vi "Main.vi"() -> ()   [LabVIEW 2014]
doc: "The boiler controller allows a user to start and shut down a boiler.\n\nUse the Reset, Start, and Light Pilot controls to sequentially start the boiler. \nUse the Fuel Control Valve to change the flow of fuel into the boiler. \nUse the Stop Boiler button to shut down the boiler. \nTo shut down the system or in the event of an emergency, use the Emergency Stop button to close the application completely."
uses:
  controls/MHL Data.ctl
  controls/MHL UI Data.ctl
  controls/MHL Status.ctl
  controls/MHL References.ctl
  controls/MHL Configuration.ctl
  support/Boiler System Globals.vi
  <vilib>/Utility/error.llb/Error Cluster From Error Code.vi
  <vilib>/ErrorRing/Error Ring.xnode
  support/Message Queue/Message Queue.lvlib
  support/User Event - Stop/User Event - Stop.lvlib
  Controller/Controller.lvlib
  Boiler/Boiler.lvlib
panel:
  in  "Fuel Control Valve":u32(slide) min=10 max=75 scale=10.0..75.0
  in  "Stop Boiler":bool
  in  "Light Pilot":bool
  out "Forced Draft Fan":bool
  out "Pilot":bool
  out "Pilot Gas Valve":bool
  out "Primary Fan":bool
  out "Status":string
  in  "Start":bool
  in  "Reset":bool
  in  "Emergency Stop":bool
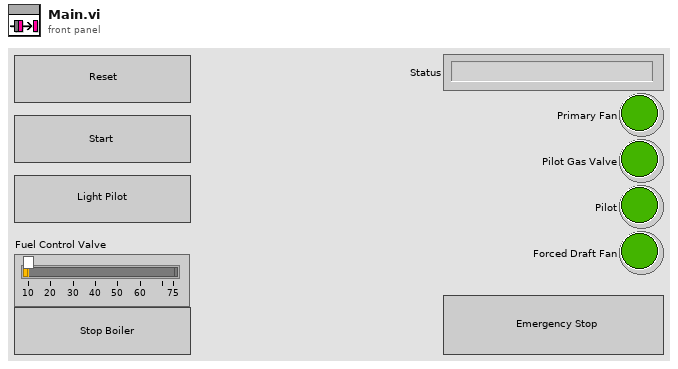
[diagram p1: front panel]
types:
  T1 = typedef "MHL Data.ctl" = cluster{"MHL User Interface Data":T2, "MHL References":T4, "MHL Configuration":T5}
  T2 = typedef "MHL UI Data.ctl" = cluster{"Status":string, "Fuel Control Valve":u32, "Primary Fan":bool, "Pilot Gas Valve":bool, "Pilot":bool, "Forced Draft Fan":bool, "MHL Status":T3}
  T3 = typedef "MHL Status.ctl" = enum16{"Lockout", "Ready", "Pre-Purge", "Pre-Purge Complete", "Pilot On", "Boiler Running", "Shutdown", "Purge"}
  T4 = typedef "MHL References.ctl" = cluster{"Reset Ref":refnum<vi>, "Start Ref":refnum<vi>, "Light Pilot Ref":refnum<vi>, "Stop Boiler Ref":refnum<vi>, "Fuel Control Valve Ref":refnum<vi>}
  T5 = typedef "MHL Configuration.ctl" = cluster{"Fuel Control Valve Maximum":dbl, "Fuel Control Valve Minimum":dbl}
  T6 = typedef "Configuration Data.ctl" = cluster{"MHL Configuration":T5, "Controller Configuration":T7, "Boiler Configuration":T8}
  T7 = typedef "Controller.lvlib/Controller Configuration.ctl" = cluster{"Purge Time":u32, "Flame Threshold":u32}
  T8 = typedef "Boiler.lvlib/Boiler Configuration.ctl" = cluster{"Pilot Increment (ms)":u32, "Pilot Decrement (ms)":u32}
  T9 = typedef "Notifiers.ctl" = cluster{"Handshake":refnum<notifier>, "Flame Level":refnum<notifier>, "Controller Exit":refnum<notifier>, "Boiler Exit":refnum<notifier>}
  T10 = typedef "Message Queue.lvlib/All Message Queues.ctl" = cluster{"MHL":refnum<queue>, "Boiler Controller":refnum<queue>, "Boiler":refnum<queue>}
  T11 = enum16{"open", "replace", "create", "open or create", "replace or create", "replace or create with confirmation"}
  T12 = enum32{"invalid app kind", "Development System", "Run Time System", "Student Edition", "Embedded LabVIEW", "Evaluation", "Custom"}
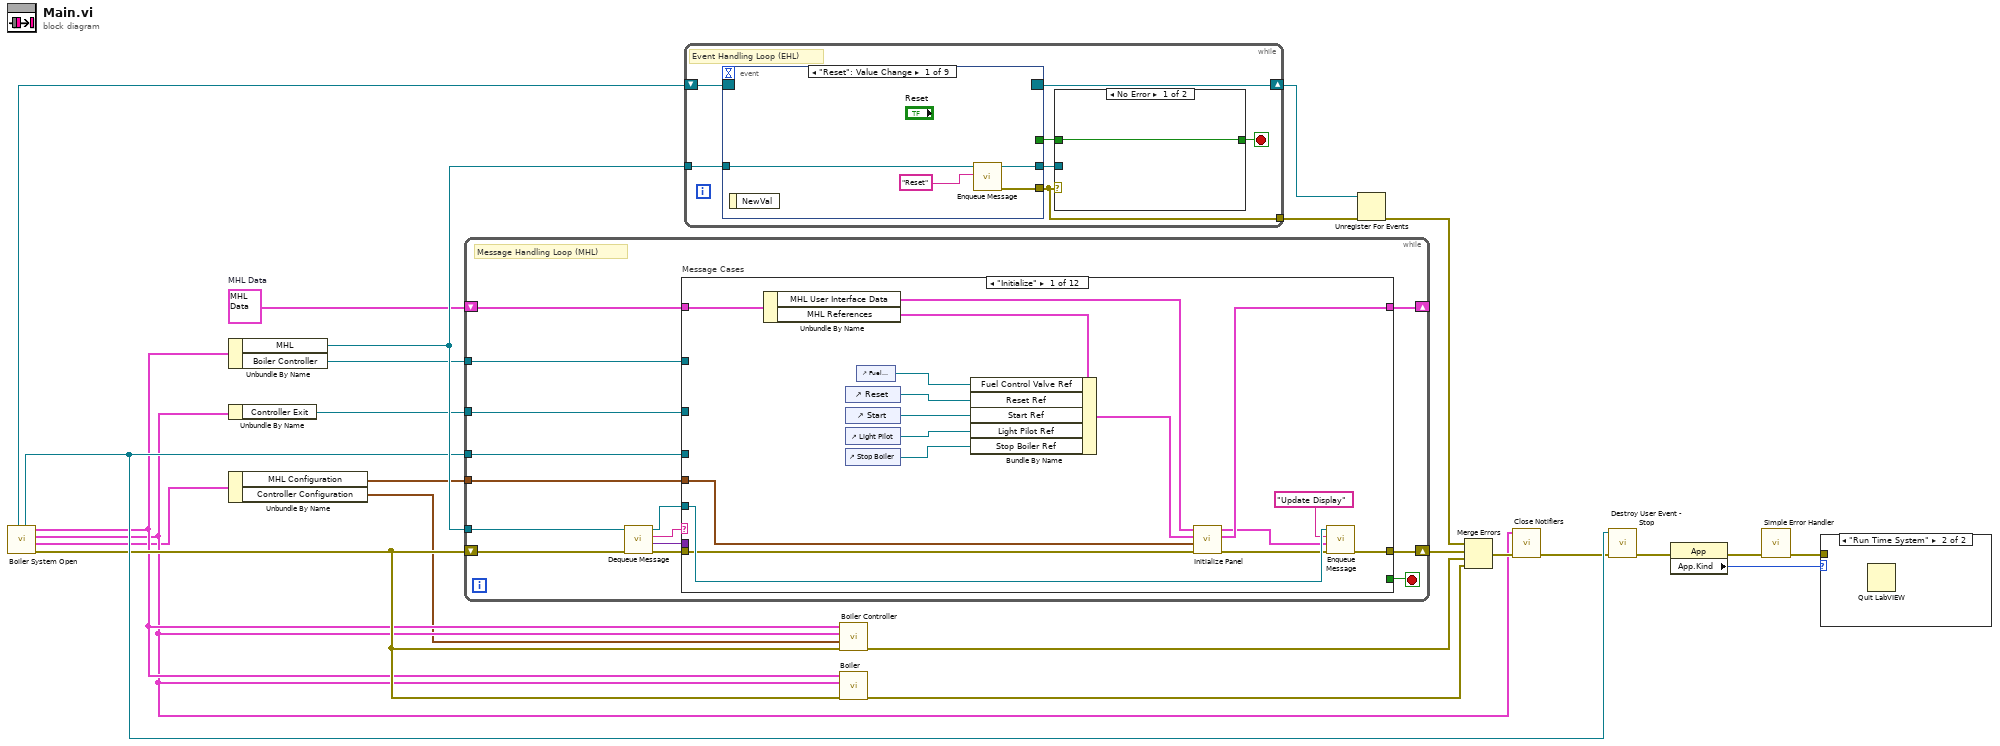
[diagram p0: block diagram]
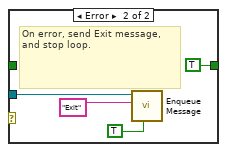
[diagram p3: hidden frame]
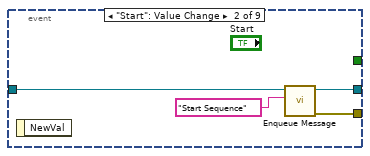
[diagram p4: hidden frame]
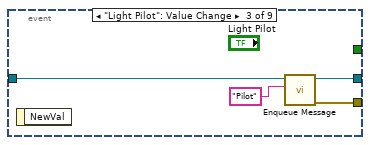
[diagram p5: hidden frame]
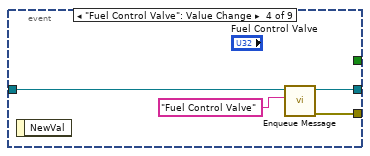
[diagram p6: hidden frame]
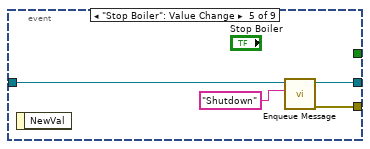
[diagram p7: hidden frame]
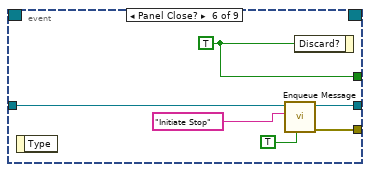
[diagram p8: hidden frame]
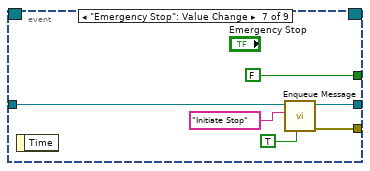
[diagram p9: hidden frame]
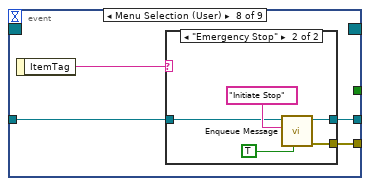
[diagram p10: hidden frame]
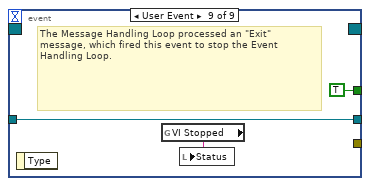
[diagram p12: hidden frame]
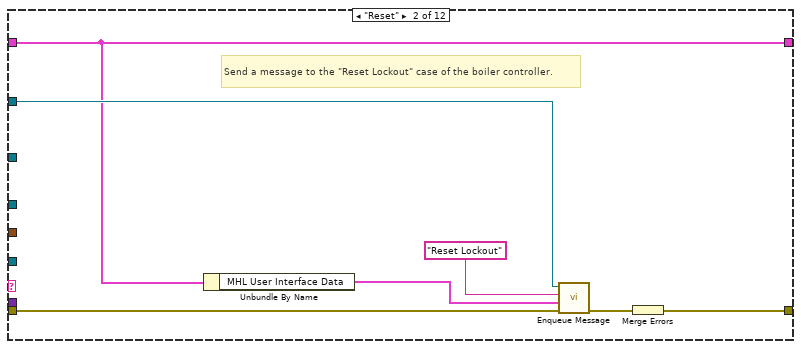
[diagram p13: hidden frame]
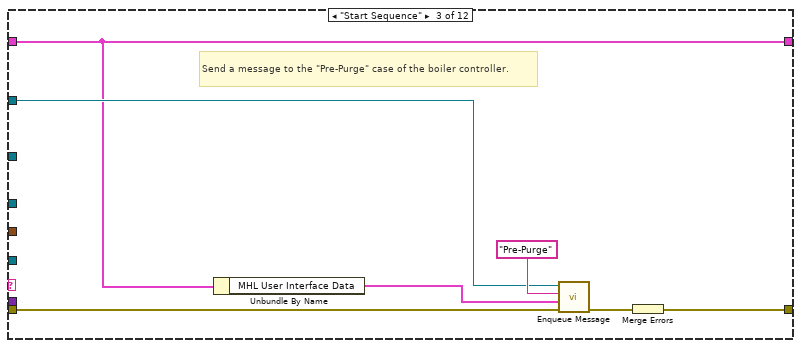
[diagram p14: hidden frame]
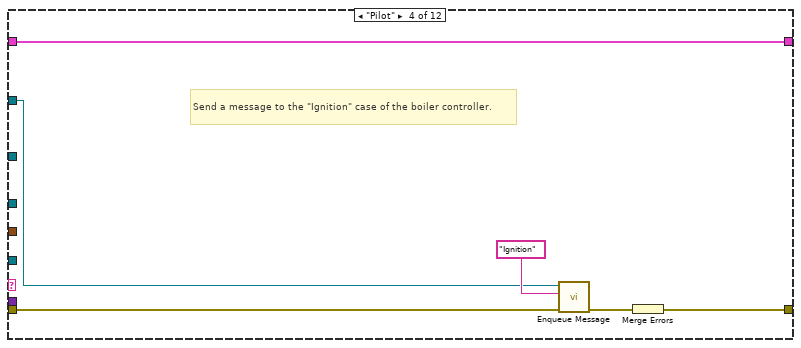
[diagram p15: hidden frame]
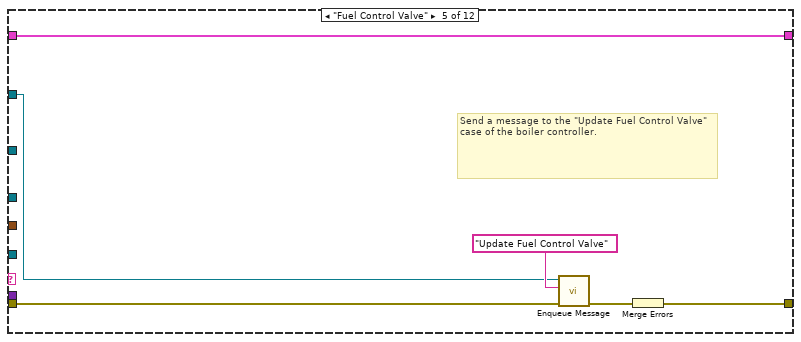
[diagram p16: hidden frame]
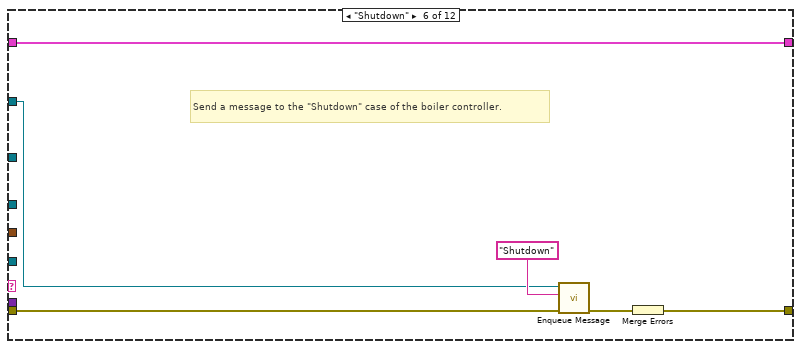
[diagram p17: hidden frame]
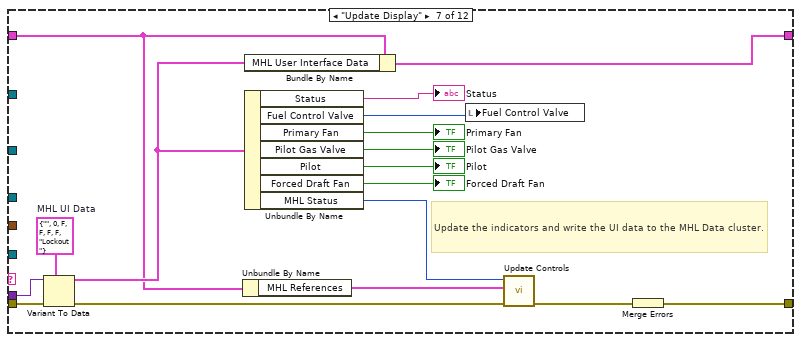
[diagram p18: hidden frame]
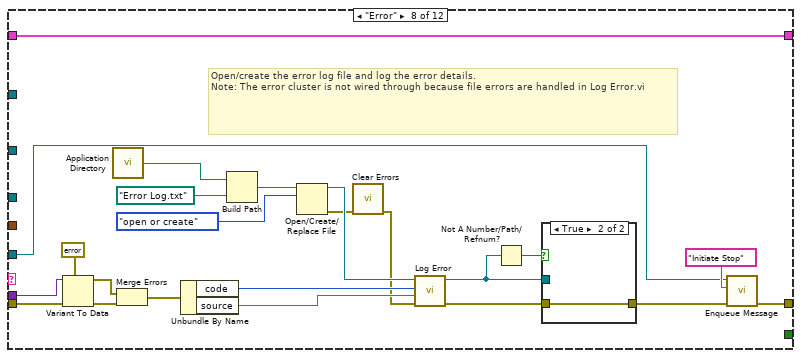
[diagram p19: hidden frame]
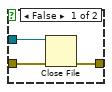
[diagram p20: hidden frame]
diagram:
  w18 = T1 {"MHL User Interface Data"={"Status"="", "Fuel Control Valve"=0, "Primary Fan"=FALSE, "Pilot Gas Valve"=FALSE, "Pilot"=FALSE, "Forced Draft Fan"=FALSE, "MHL Status"=enum."Lockout"}, "MHL References"={"Reset Ref"=refnum, "Start Ref"=refnum, "Light Pilot Ref"=refnum, "Stop Boiler Ref"=refnum, "Fuel Control Valve Ref"=refnum}, "MHL Configuration"={"Fuel Control Valve Maximum"=0.0, "Fuel Control Valve Minimum"=0.0}}  # MHL Data
  n1 = call "Boiler System Open.vi"() -> ("error out"=w9:errorcluster, "Configuration Data"=w3:T6, "Notifiers"=w4:T9, "Message Queues"=w8:T10, "User Event - Stop"=w11:refnum<user-event>, "Stop Event Registration Refnum"=w12:refnum<event-registration>)  [unwired: 6 in]
  n2 = Unbundle By Name(w8) -> ("MHL"=w23:refnum<queue>, "Boiler Controller"=w16:refnum<queue>)
  n3 = Unbundle By Name(w4) -> ("Controller Exit"=w10:refnum<notifier>)
  n4 = Unbundle By Name(w3) -> ("MHL Configuration"=w2:T5, "Controller Configuration"=w1:T7)
  n5 = while {
    tunnel: w23 -> [w28]
    shift-right: [w37] -> _
    shift-left: w18 -> [w38]
    tunnel: w11 -> [w34]
    shift-right: [w35] -> w24
    shift-left: w9 -> [w33]
    tunnel: w16 -> [w27]
    tunnel: w10 -> [w26]
    tunnel: w2 -> [w25]
    stop <- w36 stop-if-true
    # "Message Handling Loop (MHL)"
    n6 = call "Dequeue Message.vi"("error in (no error)"=w33, "Message Queue"=w28) -> ("error out"=w32:errorcluster, "Message Data"=w30:variant, "Message"=w31:string, "dup Message Queue"=w29:refnum<queue>)  [unwired: 6 in]
    n7 = case "Message Cases" shown="\"Initialize\"" w31 {
      selector: w31 -> [_ _ _ _ _ _ _ _ _ _ _ w165]
      tunnel: w29 -> [w48 _ _ _ _ _ _ w113 w134 w141 w163 _]
      tunnel: w32 -> [w42 w61 w68 w73 w76 w85 w103 w111 w139 w143 w156 _]
      tunnel: [w49 w62 w69 w74 w81 w86 w104 w109 w136 w142 w159 w164] -> w35
      tunnel: w38 -> [w50 w57 w64 w75 w77 w87 w89 w127 w138 w147 w162 w166]
      tunnel: [w40 w57 w64 w75 w77 w87 w93 w127 w138 w147 w162 w166] -> w37
      tunnel: [_ _ _ _ _ _ _ _ _ _ TRUE _] -> w36
      tunnel: w30 -> [_ _ _ _ _ _ w102 w110 _ _ _ _]
      tunnel: w34 -> [_ _ _ _ _ _ _ _ _ _ w158 _]
      tunnel: w27 -> [_ w58 w65 w70 w78 w82 _ _ w135 _ _ _]
      tunnel: w26 -> [_ _ _ _ _ _ _ _ _ w140 _ _]
      tunnel: w25 -> [w46 _ _ _ _ _ _ _ _ _ _ _]
      frame "Initialize" {
        n8 = Unbundle By Name(w50) -> ("MHL User Interface Data"=w43:T2, "MHL References"=w44:T4)
        n9 = control-ref of="Reset"() -> (w52:refnum<vi>)
        n10 = control-ref of="Start"() -> (w53:refnum<vi>)
        n11 = control-ref of="Light Pilot"() -> (w54:refnum<vi>)
        n12 = control-ref of="Stop Boiler"() -> (w55:refnum<vi>)
        n13 = control-ref of="Fuel Control Valve"() -> (w51:refnum<vi>)
        n14 = Bundle By Name(cluster=w44, "Fuel Control Valve Ref"=w51, "Reset Ref"=w52, "Start Ref"=w53, "Light Pilot Ref"=w54, "Stop Boiler Ref"=w55) -> (w45:T4)
        n15 = call "Initialize Panel.vi"("error in"=w42, "MHL Configuration"=w46, "MHL References"=w45, "MHL UI Data in"=w43) -> ("error out"=w41:errorcluster, "MHL Data out"=w40:T1, "MHL UI Data out"=w39:T2)  [unwired: 5 in]
        n16 = call "Enqueue Message.vi"("error in (no error)"=w41, "Message Data"=w39, "Message"="Update Display", "Message Queue"=w48) -> ("error out"=w49:errorcluster)  [unwired: 6 in, 1 out]
      }
      frame "Reset" {
        # "Send a message to the \"Reset Lockout\" case of the boiler controller."
        n17 = Unbundle By Name(w57) -> ("MHL User Interface Data"=w56:T2)
        n18 = call "Enqueue Message.vi"("error in (no error)"=w61, "Message Data"=w56, "Message"="Reset Lockout", "Message Queue"=w58) -> ("error out"=w60:errorcluster)  [unwired: 6 in, 1 out]
        n19 = Merge Errors(w60) -> (w62:errorcluster)
      }
      frame "Start Sequence" {
        # "Send a message to the \"Pre-Purge\" case of the boiler controller."
        n20 = Unbundle By Name(w64) -> ("MHL User Interface Data"=w63:T2)
        n21 = call "Enqueue Message.vi"("error in (no error)"=w68, "Message Data"=w63, "Message"="Pre-Purge", "Message Queue"=w65) -> ("error out"=w67:errorcluster)  [unwired: 6 in, 1 out]
        n22 = Merge Errors(w67) -> (w69:errorcluster)
      }
      frame "Pilot" {
        # "Send a message to the \"Ignition\" case of the boiler controller."
        n23 = call "Enqueue Message.vi"("error in (no error)"=w73, "Message"="Ignition", "Message Queue"=w70) -> ("error out"=w72:errorcluster)  [unwired: 7 in, 1 out]
        n24 = Merge Errors(w72) -> (w74:errorcluster)
      }
      frame "Fuel Control Valve" {
        # "Send a message to the \"Update Fuel Control Valve\" case of the boiler controller."
        n25 = call "Enqueue Message.vi"("error in (no error)"=w76, "Message"="Update Fuel Control Valve", "Message Queue"=w78) -> ("error out"=w80:errorcluster)  [unwired: 7 in, 1 out]
        n26 = Merge Errors(w80) -> (w81:errorcluster)
      }
      frame "Shutdown" {
        # "Send a message to the \"Shutdown\" case of the boiler controller."
        n27 = call "Enqueue Message.vi"("error in (no error)"=w85, "Message"="Shutdown", "Message Queue"=w82) -> ("error out"=w84:errorcluster)  [unwired: 7 in, 1 out]
        n28 = Merge Errors(w84) -> (w86:errorcluster)
      }
      frame "Update Display" {
        w101 = T2 {"Status"="", "Fuel Control Valve"=0, "Primary Fan"=FALSE, "Pilot Gas Valve"=FALSE, "Pilot"=FALSE, "Forced Draft Fan"=FALSE, "MHL Status"=enum."Lockout"}  # MHL UI Data
        # "Update the indicators and write the UI data to the MHL Data cluster."
        n29 = Variant To Data(error in=w103, type=w101, Variant=w102) -> (data=w94:T2, error out=w92:errorcluster)
        n30 = Unbundle By Name(w89) -> ("MHL References"=w88:T4)
        n31 = Bundle By Name(cluster=w89, "MHL User Interface Data"=w94) -> (w93:T1)
        n32 = Unbundle By Name(w94) -> ("Status"=→"Status":string, "Fuel Control Valve"=w99:u32, "Primary Fan"=→"Primary Fan":bool, "Pilot Gas Valve"=→"Pilot Gas Valve":bool, "Pilot"=→"Pilot":bool, "Forced Draft Fan"=→"Forced Draft Fan":bool, "MHL Status"=w90:T3)
        n33 = local write "Fuel Control Valve"(w99) -> ()
        n34 = call "Update Controls.vi"("error in"=w92, "MHL References"=w88, "MHL Status"=w90) -> ("error out"=w91:errorcluster)  [unwired: 8 in]
        n35 = Merge Errors(w91) -> (w104:errorcluster)
      }
      frame "Error" {
        # "Open/create the error log file and log the error details.\nNote: The error cluster is not wired through because file errors are handled in Log Error.vi"
        n36 = Variant To Data(error in=w111, type=errorcluster {"status"=FALSE, "code"=0, "source"=""} ("error out"), Variant=w110) -> (data=w123:errorcluster, error out=w124:errorcluster)
        n37 = call <vilib>:"Application Directory.vi"() -> ("Application Directory"=w121:path)
        n38 = Merge Errors(w123, w124) -> (w122:errorcluster)
        n39 = Unbundle By Name(w122) -> ("code"=w116:i32, "source"=w115:string)
        n40 = Build Path(base path=w121, name or relative path=path "Error Log.txt") -> (appended path=w120:path)
        n41 = Open/Create/Replace File(file path (use dialog)=w120, operation (0:open)=T11."open or create") -> (refnum out=w118:refnum<file>, error out=w106:errorcluster)  [unwired: 4 in, 1 out]
        n42 = call <vilib>:"Clear Errors.vi"("error in (no error)"=w106) -> ("error out"=w105:errorcluster)  [unwired: 5 in, 1 out]
        n43 = call "Log Error.vi"("error in"=w105, "Source"=w115, "Code"=w116, "Error Log Refnum In"=w118) -> ("error out"=w117:errorcluster, "Error Log Refnum Out"=w108:refnum<file>)  [unwired: 6 in]
        n44 = Not A Number/Path/Refnum?(number/path/refnum=w108) -> (NaN/Path/Refnum?=w107:bool)
        n45 = case shown="True" w107 {
          tunnel: w117 -> [w130 w131]
          tunnel: w108 -> [w129 _]
          tunnel: [w128 w131] -> w114
          frame False {
            n46 = Close File(refnum=w129, error in=w130) -> (error out=w128:errorcluster)  [unwired: 1 out]
          }
          frame True {
          }
        }
        n47 = call "Enqueue Message.vi"("error in (no error)"=w114, "Message"="Initiate Stop", "Message Queue"=w113) -> ("error out"=w109:errorcluster)  [unwired: 7 in, 1 out]
      }
      frame "Initiate Stop" {
        # "When stopping, first send a message to stop the boiler controller. Then wait for the boiler and boiler controller to exit."
        n48 = call "Enqueue Message.vi"("error in (no error)"=w139, "Message"="Exit", "Message Queue"=w135) -> ("error out"=w137:errorcluster)  [unwired: 7 in, 1 out]
        n49 = call "Enqueue Message.vi"("error in (no error)"=w137, "Message"="Wait on Boiler Exit", "Message Queue"=w134) -> ("error out"=w136:errorcluster)  [unwired: 7 in, 1 out]
      }
      frame "Wait on Boiler Exit" {
        # "Monitor the boiler controller to determine if it has completed its Exit. Wait 10 milliseconds for the boiler controller to respond. \nIf the notification does not occur, then enqueue another Wait on Boiler Exit message.\nIf the notification occurs, then exit the Message Handling Loop."
        n50 = Wait on Notification(notifier=w140, timeout in ms (-1)=10, error in (no error)=w143) -> (timed out?=w145:bool, error out=w144:errorcluster)  [unwired: 1 in, 2 out]
        n51 = case shown="True" w145 {
          tunnel: w144 -> [w151 w155]
          tunnel: w141 -> [w150 w153]
          tunnel: [w148 w154] -> w142
          frame False {
            n52 = call "Enqueue Message.vi"("error in (no error)"=w151, "Message"="Exit", "Message Queue"=w150) -> ("error out"=w148:errorcluster)  [unwired: 7 in, 1 out]
          }
          frame True {
            n53 = call "Enqueue Message.vi"("error in (no error)"=w155, "Message"="Wait on Boiler Exit", "Message Queue"=w153) -> ("error out"=w154:errorcluster)  [unwired: 7 in, 1 out]
          }
        }
      }
      frame "Exit" {
        # "Stop the VI"
        # "Release the message queue reference"
        n54 = call "Fire User Event - Stop.vi"("User Event - Stop"=w158) -> ("error out"=w157:errorcluster)  [unwired: 10 in]
        n55 = Release Queue(queue=w163, error in (no error)=w156) -> (error out=w160:errorcluster)  [unwired: 1 in, 2 out]
        n56 = Merge Errors(w157, w160) -> (w159:errorcluster)
      }
      frame Default {
        # "'Default' case only runs if there is a message that isn't defined in any of the other cases.  Output a programming error."
        n57 = xnode "Error Ring"("parameter 0"=w165) -> ("error out"=w164:errorcluster)
      }
    }
  }
  n58 = while {
    tunnel: w23 -> [w180]
    tunnel: [w176] -> w20
    shift-right: [w174] -> w19
    shift-left: w12 -> [w175]
    stop <- w178 stop-if-true
    # "Event Handling Loop (EHL)"
    n59 = event shown="[0] \"Reset\": Value Change" {
      selector: w175 -> [_ _ _ _ _ _ _ _ _]
      dyn-events: [_ _ _ _ _ _ _ _ _] -> w174
      timeout: _ -> [_ _ _ _ _ _ _ _ _]
      tunnel: [_ _ _ _ _ w211 FALSE ("Discard?") _ TRUE ("Discard?")] -> w179
      tunnel: w180 -> [w189 w193 w197 w201 w205 w210 w217 w220 w230]
      tunnel: [w188 w191 w195 w199 w203 w209 w216 w218 _] -> w176
      tunnel: [w187 w192 w196 w200 w204 w208 w214 w219 w230] -> w177
      event "Reset": Value Change {
        n60 = event-data() -> ()  [unwired: 1 in, 1 out]
        n61 = call "Enqueue Message.vi"("Message"="Reset", "Message Queue"=w189) -> ("error out"=w188:errorcluster, "dup Message Queue"=w187:refnum<queue>)  [unwired: 8 in]
      }
      event "Start": Value Change {
        n62 = event-data() -> ()  [unwired: 1 in, 1 out]
        n63 = call "Enqueue Message.vi"("Message"="Start Sequence", "Message Queue"=w193) -> ("error out"=w191:errorcluster, "dup Message Queue"=w192:refnum<queue>)  [unwired: 8 in]
      }
      event "Light Pilot": Value Change {
        n64 = event-data() -> ()  [unwired: 1 in, 1 out]
        n65 = call "Enqueue Message.vi"("Message"="Pilot", "Message Queue"=w197) -> ("error out"=w195:errorcluster, "dup Message Queue"=w196:refnum<queue>)  [unwired: 8 in]
      }
      event "Fuel Control Valve": Value Change {
        n66 = event-data() -> ()  [unwired: 1 in, 1 out]
        n67 = call "Enqueue Message.vi"("Message"="Fuel Control Valve", "Message Queue"=w201) -> ("error out"=w199:errorcluster, "dup Message Queue"=w200:refnum<queue>)  [unwired: 8 in]
      }
      event "Stop Boiler": Value Change {
        n68 = event-data() -> ()  [unwired: 1 in, 1 out]
        n69 = call "Enqueue Message.vi"("Message"="Shutdown", "Message Queue"=w205) -> ("error out"=w203:errorcluster, "dup Message Queue"=w204:refnum<queue>)  [unwired: 8 in]
      }
      event Panel Close? {
        w211 = TRUE ("Discard?")
        n70 = event-data() -> ()  [unwired: 1 in, 1 out]
        n71 = call "Enqueue Message.vi"("Priority Message? (F)"=TRUE, "Message"="Initiate Stop", "Message Queue"=w210) -> ("error out"=w209:errorcluster, "dup Message Queue"=w208:refnum<queue>)  [unwired: 7 in]
        n72 = event-data("Discard?"=w211) -> ()  [unwired: 1 in, 1 out]
      }
      event "Emergency Stop": Value Change {
        n73 = event-data() -> ()  [unwired: 1 in, 1 out]
        n74 = call "Enqueue Message.vi"("Priority Message? (F)"=TRUE, "Message"="Initiate Stop", "Message Queue"=w217) -> ("error out"=w216:errorcluster, "dup Message Queue"=w214:refnum<queue>)  [unwired: 7 in]
      }
      event Menu Selection (User) {
        n75 = event-data() -> ("ItemTag"=w221:string)  [unwired: 1 in]
        n76 = case shown="\"Emergency Stop\"" w221 {
          tunnel: w220 -> [w222 w225]
          tunnel: [w222 w224] -> w219
          tunnel: [_ w223] -> w218
          frame Default {
          }
          frame "Emergency Stop" {
            n77 = call "Enqueue Message.vi"("Priority Message? (F)"=TRUE, "Message"="Initiate Stop", "Message Queue"=w225) -> ("error out"=w223:errorcluster, "dup Message Queue"=w224:refnum<queue>)  [unwired: 7 in]
          }
        }
      }
      event User Event {
        # "The Message Handling Loop processed an \"Exit\" message, which fired this event to stop the Event Handling Loop."
        n78 = event-data() -> ()  [unwired: 1 in, 1 out]
        n79 = global read "Boiler System Globals.vi" "VI Stopped"() -> (w228:string)
        n80 = local write "Status"(w228) -> ()
      }
    }
    n81 = case shown="No Error" w176 {
      tunnel: [w181 TRUE ("Discard?")] -> w178
      tunnel: w179 -> [w181 _]
      tunnel: w177 -> [_ w184]
      frame No Error {
      }
      frame Error {
        # "On error, send Exit message, and stop loop."
        n82 = call "Enqueue Message.vi"("Priority Message? (F)"=TRUE, "Message"="Exit", "Message Queue"=w184) -> ()  [unwired: 7 in, 2 out]
      }
    }
  }
  n83 = call "Boiler Controller.vi"("error in"=w9, "Controller Configuration"=w1, "Notifiers"=w4, "Message Queues"=w8) -> ("error out"=w17:errorcluster)  [unwired: 7 in]
  n84 = call "Boiler.vi"("error in"=w9, "Notifiers"=w4, "Message Queues"=w8) -> ("error out"=w7:errorcluster)  [unwired: 8 in]
  n85 = Unregister For Events(event registration refnum=w19, error in=w20) -> (error out=w21:errorcluster)
  n86 = Merge Errors(w21, w24, w17, w7) -> (w6:errorcluster)
  n87 = call "Close Notifiers.vi"("error in"=w6, "Notifiers"=w4) -> ("error out"=w5:errorcluster)  [unwired: 9 in]
  n88 = call "Destroy User Event - Stop.vi"("error in (no error)"=w5, "User Event - Stop"=w11) -> ("error out"=w22:errorcluster)  [unwired: 9 in]
  n89 = property class="App"(error in=w22) -> (error out=w15:errorcluster, "App.Kind"=w14:T12)  [unwired: 1 in, 1 out]
  n90 = call <vilib>:"Simple Error Handler.vi"("error in (no error)"=w15) -> ("error out"=w13:errorcluster)  [unwired: 4 in, 4 out]
  n91 = case shown="\"Run Time System\"" w14 {
    tunnel: w13 -> [_ _]
    frame Default {
    }
    frame "Run Time System" {
      n92 = Quit LabVIEW() -> ()  [unwired: 1 in]
    }
  }
